vi "Signal Level & Frequency.vi"(5 "Frequency Value (Hz) (100KHz)":dbl=100000.0 min=20.0 max=30000000.0 step=1.0 format="%.4f", 6 "Oscillator Select (T: Voltage)":bool=TRUE, 7 "Current Level (A) (100uA)":dbl=0.0001 min=0.0001 max=20.0 step=0.01 format="%.4f", 8 "error in (no error)":errorcluster, 9 "Voltage Level (V) (5mV)":dbl=0.005 min=0.005 max=20.0 step=0.001 format="%.4f", 10 "Auto Level Control (F: Off)":bool, 11 "VISA resource name":refnum<visa-resource-name>) -> (0 "error out":errorcluster, 3 "VISA resource name out":refnum<visa-resource-name>)   [LabVIEW 2015, in "Agilent 428X Series.lvlib"]
doc: "This function sets the oscillator's output voltage/current level, frequency and switch ON/OFF Automatic Level Control (ALC)."
uses:
  Agilent 428X Series.lvlib
panel:
  # "On\nOff"
  # "Voltage\nCurrent"
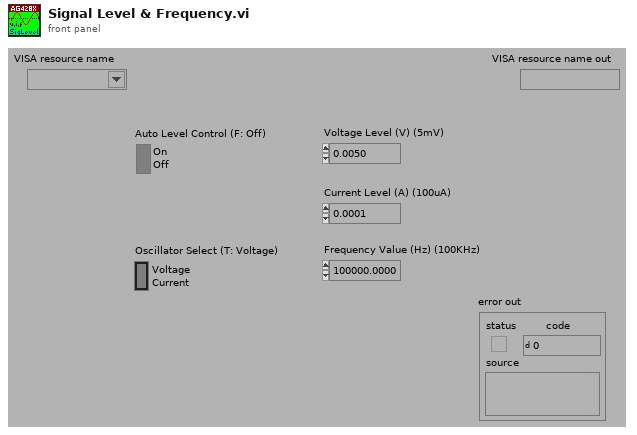
[diagram p1: front panel]
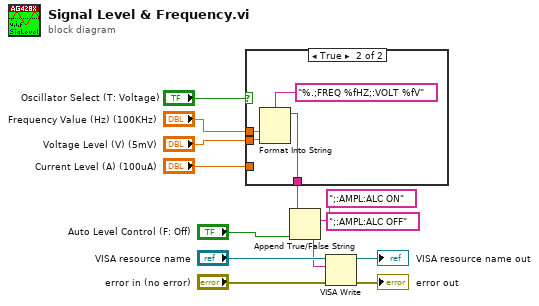
[diagram p0: block diagram]
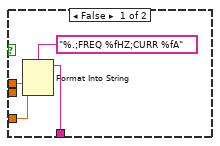
[diagram p2: hidden frame]
diagram:
  n1 = case shown="True" "Oscillator Select (T: Voltage)" {
    tunnel: [w17 w21] -> w10
    tunnel: "Voltage Level (V) (5mV)" -> [_ w18]
    tunnel: "Frequency Value (Hz) (100KHz)" -> [w15 w19]
    tunnel: "Current Level (A) (100uA)" -> [w14 _]
    frame False {
      n2 = Format Into String(format string="%.;FREQ %fHZ;CURR %fA", w15, w14) -> (resulting string=w17:string)  [unwired: 2 in, 1 out]
    }
    frame True {
      n3 = Format Into String(format string="%.;FREQ %fHZ;:VOLT %fV", w19, w18) -> (resulting string=w21:string)  [unwired: 2 in, 1 out]
    }
  }
  n4 = Append True/False String(1:"Auto Level Control (F: Off)", 2:";:AMPL:ALC OFF" ("true string"), 3:";:AMPL:ALC ON" ("true string"), 4:w10) -> (0:w3:string)
  n5 = VISA Write(VISA resource name="VISA resource name", write buffer=w3, error in (no error)="error in (no error)") -> (VISA resource name out=→"VISA resource name out":refnum<visa-resource-name>, error out=→"error out":errorcluster)  [unwired: 1 out]
